vi "图像采集与保存-原版.vi"(9 "Grab":bool, 10 "保存图像":bool, 11 "Camera Name":refnum<k21>="cam0" caption="IMAQdx Session") -> ()   [LabVIEW 2018]
doc: "The Grab and Attributes Setup example VI allows the user to view the current attributes and settings, update attribute settings, acquire images continuously, and display the images in an image control."
uses:
  <vilib>/vision/driver/IMAQdx.llb/IMAQdx Acquisition Mode.ctl
  <vilib>/vision/driver/IMAQdx.llb/IMAQdx Buffer Number Mode.ctl
  <vilib>/vision/driver/NI_Vision_Acquisition_Software.lvlib
panel:
  in  "确定按钮":bool
  in  "Tab Control":T1(tab)
  in  "U32 Value Control":u32(slide) min=1 step=1 scale=1.0..4294967295.0
  in  "DBL Value Control":dbl(slide) min=2.2571161239684447 max=1000.0 step=1.0 scale=2.2571161239684447..1000.0
  in  "String Value Control":string
  in  "Enum Value Control":u32(ring) items=["Unicast", "Broadcast", "Multicast"]
  in  "Boolean Value Control":bool
  in  "Command Value Control":bool
  out "Tooltip":string="Gets/Sets the maximum number of outstanding events to queue."
  out "Units":string
  in  "Attribute Tree":string(tree)
  out "Frame Rate":dbl(knob) scale=0.0..100.0
  out "Image":T2(plugin-control)
  out "Buffer Number":u32
  in  "Stop":bool
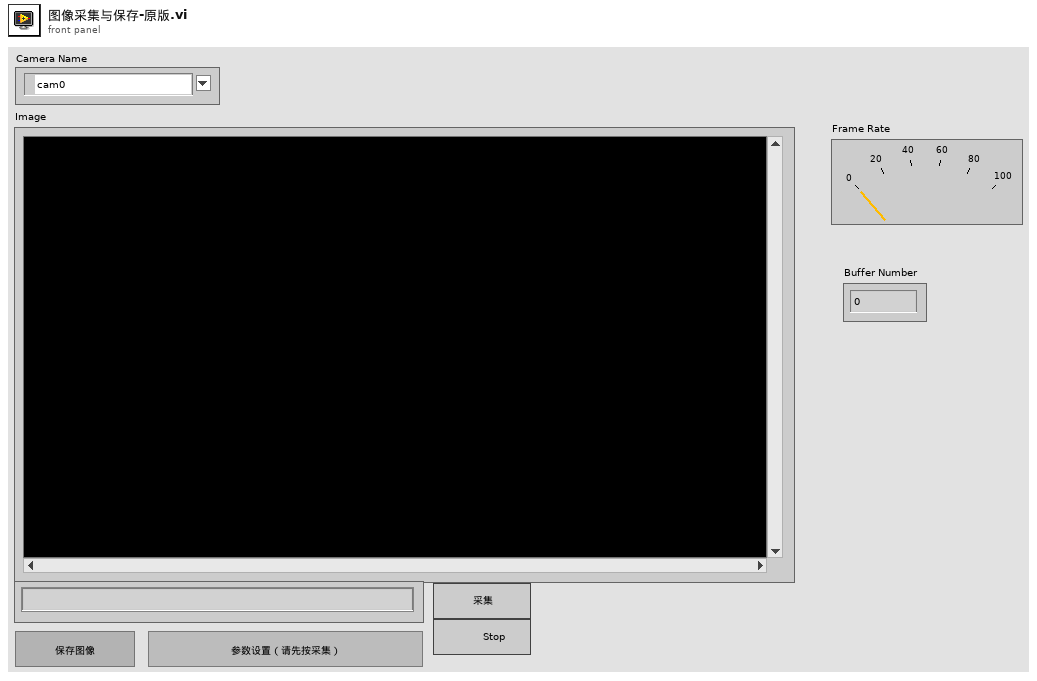
[diagram p1: front panel]
types:
  T1 = enum32{"U32", "DBL", "String", "Enum", "Bool", "Command"}
  T2 = typedef "IMAQ Image.ctl" = refnum<image>
  T3 = typedef "NI_Vision_Acquisition_Software.lvlib/IMAQdx Acquisition Mode.ctl" = enum32{"One Shot", "Continuous"}
  T4 = typedef "IMAQdx.ctl" = refnum<k21>
  T5 = cluster{"Tab Control":refnum<vi>, "U32 Value Control":refnum<vi>, "DBL Value Control":refnum<vi>, "String Value Control":refnum<vi>, "Enum Value Control":refnum<vi>, "Boolean Value Control":refnum<vi>, "Command Value Control":refnum<vi>}
  T6 = typedef "NI_Vision_Acquisition_Software.lvlib/IMAQdx Buffer Number Mode.ctl" = enum32{"Next", "Last", "Buffer Number", "Every", "Last New"}
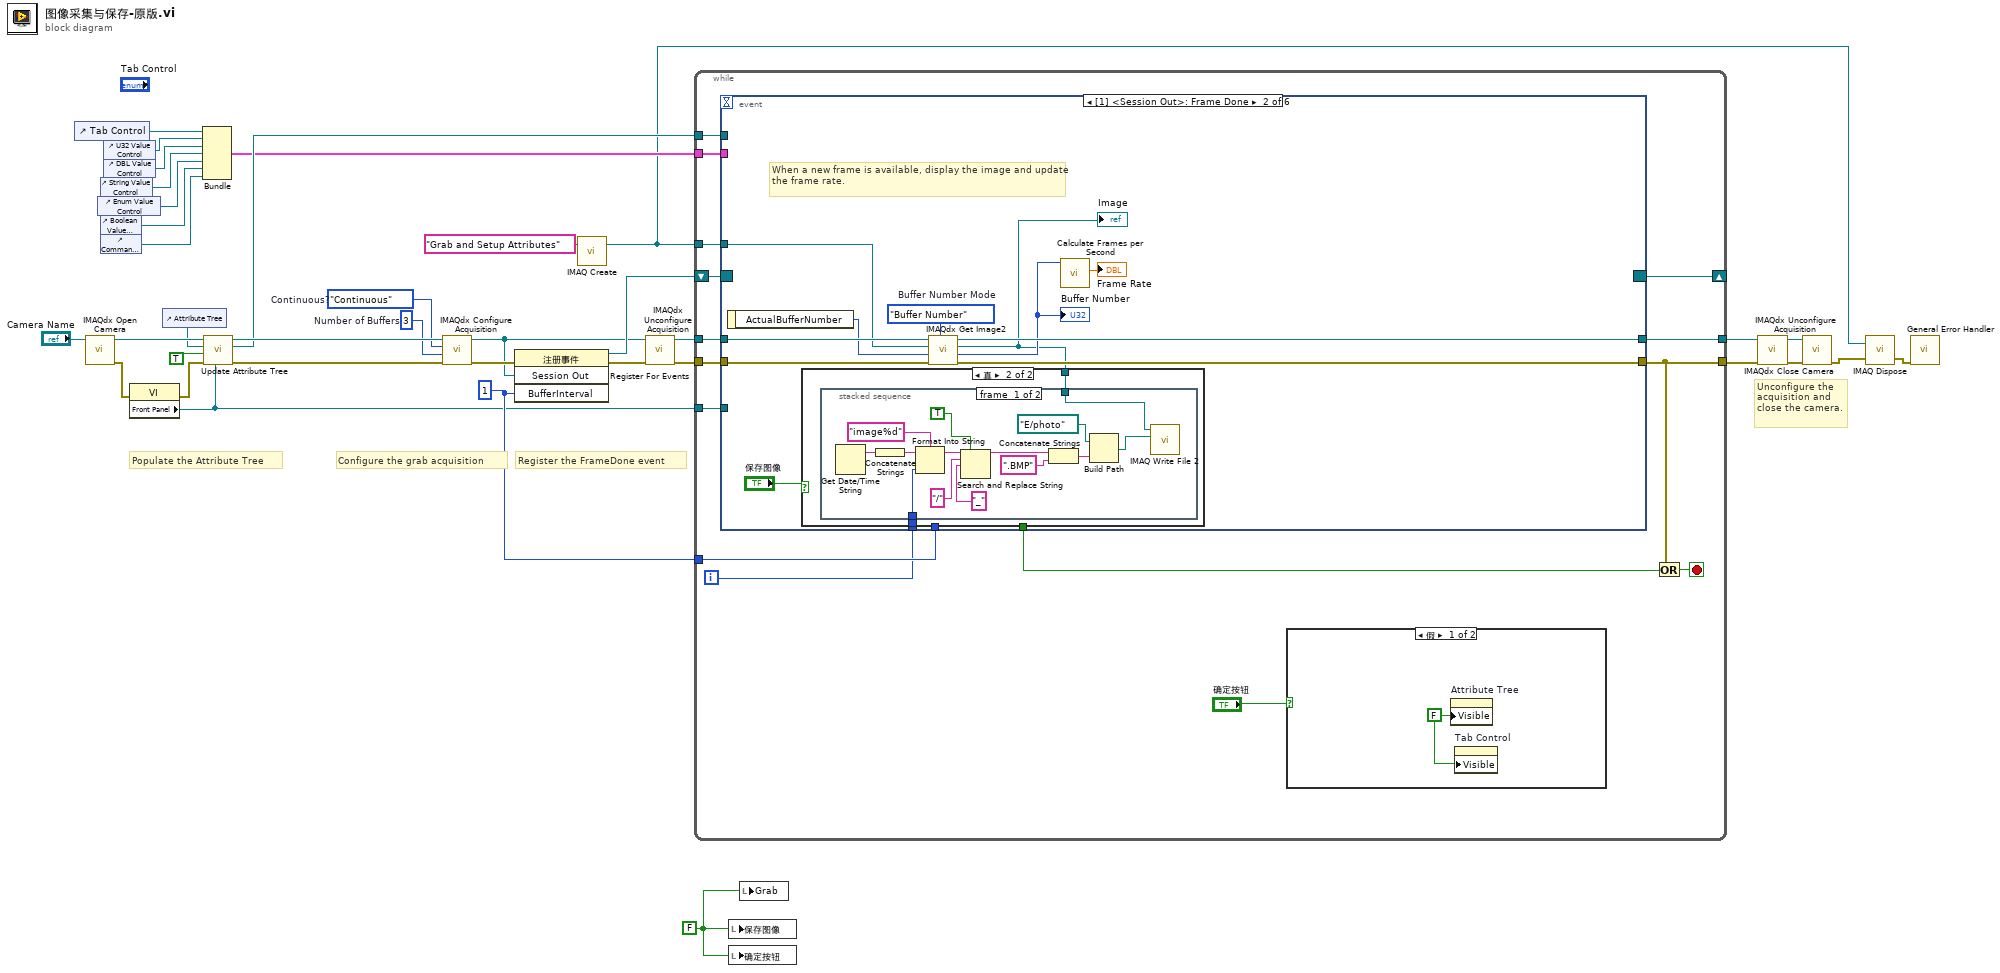
[diagram p0: block diagram]
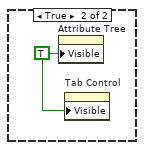
[diagram p2: hidden frame]
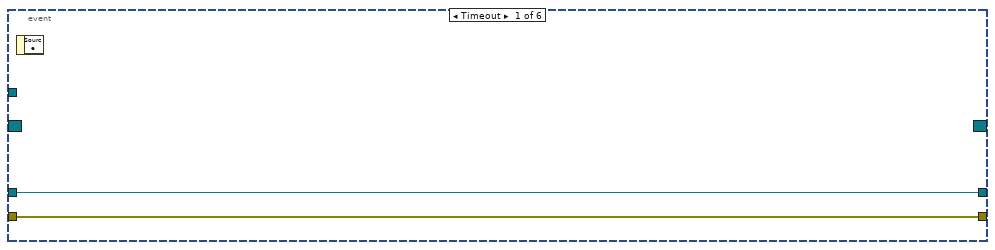
[diagram p3: hidden frame]
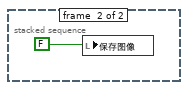
[diagram p5: hidden frame]
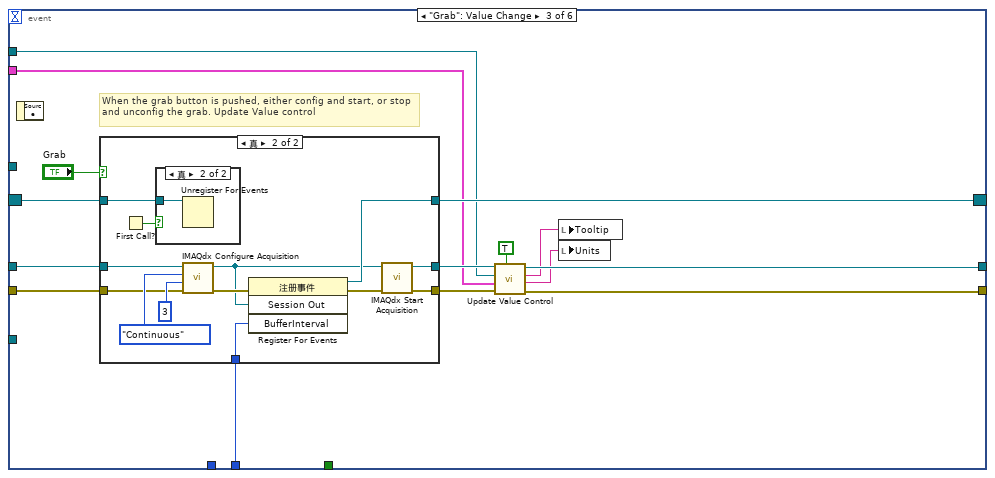
[diagram p6: hidden frame]
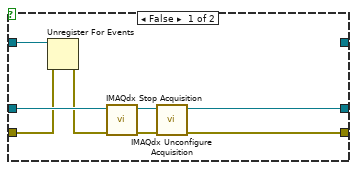
[diagram p7: hidden frame]
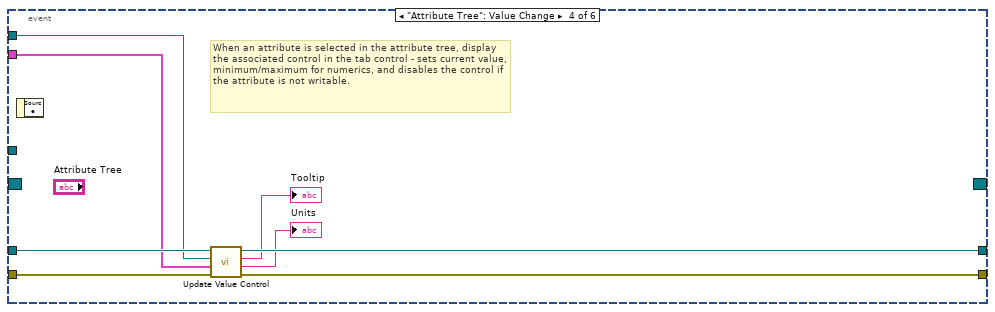
[diagram p9: hidden frame]
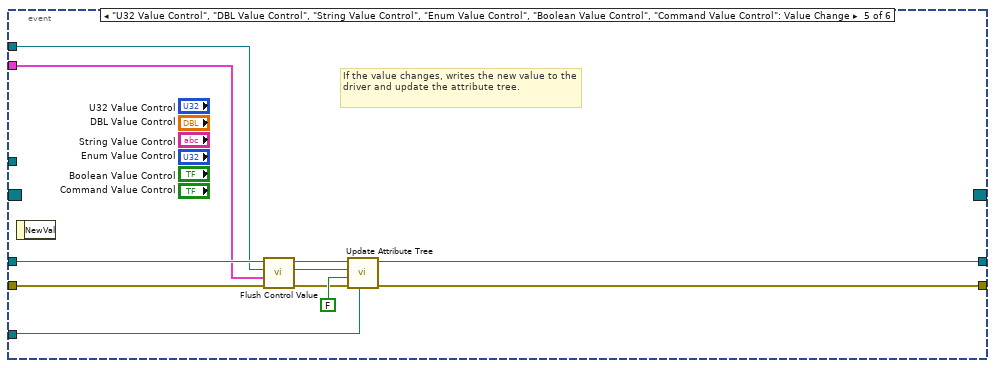
[diagram p10: hidden frame]
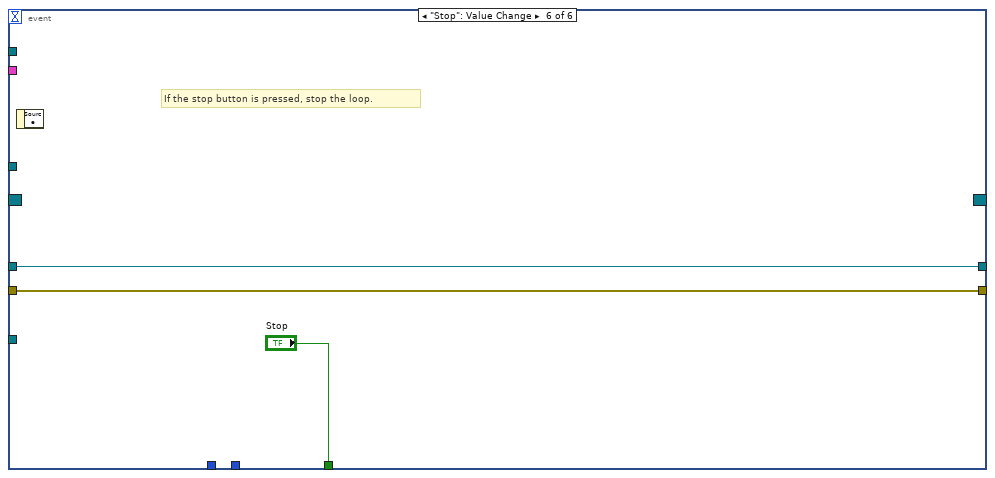
[diagram p11: hidden frame]
diagram:
  w1 = FALSE
  w17 = u32 1 ("BufferInterval")
  w3 = u32 3  # Number of Buffers
  w2 = IMAQdx_Acquisition_Mode."Continuous"  # Continuous?
  # "Unconfigure the acquisition and close the camera."
  # "Register the FrameDone event"
  # "Configure the grab acquisition"
  # "Populate the Attribute Tree"
  n1 = control-ref of="Tab Control"() -> (w7:refnum<vi>)
  n2 = call <vilib>:"IMAQdx Open Camera.vi"("Session In"="Camera Name") -> ("error out"=w20:errorcluster, "Session Out"=w25:T4)  [unwired: 2 in, 7 out]
  n3 = control-ref of="Enum Value Control"() -> (w28:refnum<vi>)
  n4 = control-ref of="String Value Control"() -> (w31:refnum<vi>)
  n5 = control-ref of="Boolean Value Control"() -> (w27:refnum<vi>)
  n6 = control-ref of="Command Value Control"() -> (w26:refnum<vi>)
  n7 = control-ref of="U32 Value Control"() -> (w30:refnum<vi>)
  n8 = control-ref of="DBL Value Control"() -> (w29:refnum<vi>)
  n9 = property class="VI"(error in=w20) -> (error out=w6:errorcluster, "Front Panel"=w4:refnum<vi>)  [unwired: 1 in, 1 out]
  n10 = control-ref of="Attribute Tree"() -> (w23:refnum<vi>)
  n11 = Bundle("Tab Control"=w7, "U32 Value Control"=w30, "DBL Value Control"=w29, "String Value Control"=w31, "Enum Value Control"=w28, "Boolean Value Control"=w27, "Command Value Control"=w26) -> (w12:T5)  [unwired: 1 out]
  n12 = call "Update Attribute Tree.vi"("Panel Refnum In"=w4, "error in"=w6, "Flush Tree?"=TRUE, "Tree Control In"=w23, "Camera Name In"=w25) -> ("error out"=w5:errorcluster, "Tree Control Out"=w21:refnum<vi>, "Session Out"=w24:T4)  [unwired: 4 in]
  n13 = call <vilib>:"IMAQdx Configure Acquisition.vi"("error in"=w5, "Number of Buffers"=w3, "Continuous?"=w2, "Session In"=w24) -> ("error out"=w33:errorcluster, "Session Out"=w14:T4)  [unwired: 6 out]
  n14 = register-events(error in=w33, w14, w17) -> (reference out=w32:refnum<event-registration>, error out=w16:errorcluster)  [unwired: 1 in]
  n15 = call "IMAQ Create"("Image Name"="Grab and Setup Attributes") -> ("New Image"=w9:T2)  [unwired: 3 in, 2 out]
  n16 = call <vilib>:"IMAQdx Unconfigure Acquisition.vi"("error in"=w16, "Session In"=w14) -> ("error out"=w15:errorcluster, "Session Out"=w13:T4)  [unwired: 8 out]
  n17 = while {
    tunnel: [w47] -> w19
    tunnel: w15 -> [w49]
    tunnel: w13 -> [w50]
    tunnel: [w40] -> w18
    tunnel: w9 -> [w48]
    tunnel: w21 -> [w45]
    tunnel: w4 -> [w44]
    tunnel: w17 -> [w42]
    shift-right: [w41] -> _
    shift-left: w32 -> [w46]
    tunnel: w12 -> [w39]
    i -> [w38]
    stop <- w51 stop-if-true
    n18 = event shown="[1] <Session Out>: Frame Done" {
      selector: w46 -> [_ _ w95 _ _ _]
      dyn-events: [_ _ w97 _ _ _] -> w41
      timeout: _ -> [_ _ _ _ _ _]
      tunnel: w50 -> [w54 w67 w99 w129 w139 w141]
      tunnel: w49 -> [w55 w66 w94 w127 w140 w142]
      tunnel: w48 -> [_ w65 _ _ _ _]
      tunnel: [w54 w64 w87 w128 w135 w141] -> w47
      tunnel: [w55 w63 w91 w126 w131 w142] -> w40
      tunnel: w45 -> [_ _ w90 w124 w133 _]
      tunnel: w44 -> [_ _ _ _ w130 _]
      tunnel: [_ _ _ _ _ "Stop"] -> w43
      tunnel: w42 -> [_ _ w96 _ _ _]
      tunnel: w39 -> [_ _ w88 w125 w134 _]
      tunnel: w38 -> [_ w57 _ _ _ _]
      event Timeout {
        n19 = event-data() -> ()  [unwired: 2 out]
      }
      event event #0x0 {
        w62 = IMAQdx_Buffer_Number_Mode."Buffer Number"  # Buffer Number Mode
        # "When a new frame is available, display the image and update the frame rate."
        n20 = event-data() -> ("ActualBufferNumber"=w61:u32)  [unwired: 1 out]
        n21 = call <vilib>:"IMAQdx Get Image2.vi"("Buffer Number Mode (Next)"=w62, "error in"=w66, "Buffer Number In"=w61, "Image In"=w65, "Session In"=w67) -> ("error out"=w63:errorcluster, "Buffer Number Out"=w60:u32, "Image Out"=w56:T2, "Session Out"=w64:T4)  [unwired: 3 in]
        "Image" <- w56
        "Buffer Number" <- w60
        n22 = case shown="真" "保存图像" {
          tunnel: w57 -> [_ w69]
          tunnel: w56 -> [_ w68]
          frame False {
          }
          frame True {
            n23 = stacked-sequence {
              tunnel: w69 -> [w71 _]
              tunnel: w68 -> [w70 _]
              frame #0 {
                n24 = Get Date/Time String() -> (date string=w75:string)  [unwired: 3 in, 1 out]
                n25 = Concatenate Strings(w75) -> (w74:string)
                n26 = Format Into String(format string="image%d" ("Image Name"), initial string=w74, w71) -> (resulting string=w72:string)  [unwired: 1 in, 1 out]
                n27 = Search and Replace String(replace all?=TRUE ("替换全部？(F)"), input string=w72, search string="/" ("搜索字符串"), replace string="_" ("替换字符串(\"\")")) -> (result string=w77:string)  [unwired: 4 in, 3 out]
                n28 = Concatenate Strings(w77, ".BMP" ("字符串")) -> (w76:string)
                n29 = Build Path(base path=path "E:/photo" ("基路径"), name or relative path=w76) -> (appended path=w83:path)
                n30 = call-poly "IMAQ Write File 2"("File Path"=w83, "Image"=w70) -> ()  [unwired: 8 in, 2 out]
              }
              frame #1 {
                n31 = local write "保存图像"(FALSE) -> ()
              }
            }
          }
        }
        n32 = call <vilib>:"Calculate Frames per Second.vi"("Buffer Number"=w60) -> ("Processed Frames/s"=→"Frame Rate":dbl)  [unwired: 8 in, 2 out]
      }
      event "Grab": Value Change {
        # "When the grab button is pushed, either config and start, or stop and unconfig the grab. Update Value control"
        n33 = event-data() -> ()  [unwired: 2 out]
        n34 = case shown="真" "Grab" {
          tunnel: w99 -> [w107 w118]
          tunnel: [w104 w120] -> w93
          tunnel: [w103 w119] -> w92
          tunnel: [_ w113] -> w97
          tunnel: w96 -> [_ w111]
          tunnel: w95 -> [w102 w109]
          tunnel: w94 -> [w100 w110]
          frame False {
            n35 = Unregister For Events(event registration refnum=w102, error in=w100) -> (error out=w101:errorcluster)
            n36 = call <vilib>:"IMAQdx Stop Acquisition.vi"("error in"=w101, "Session In"=w107) -> ("error out"=w105:errorcluster, "Session Out"=w106:T4)  [unwired: 8 out]
            n37 = call <vilib>:"IMAQdx Unconfigure Acquisition.vi"("error in"=w105, "Session In"=w106) -> ("error out"=w103:errorcluster, "Session Out"=w104:T4)  [unwired: 8 out]
          }
          frame True {
            n38 = First Call?() -> (First Call?: T/F=w108:bool)
            n39 = case shown="真" w108 {
              tunnel: w109 -> [_ w121]
              frame False {
              }
              frame True {
                n40 = Unregister For Events(event registration refnum=w121) -> ()  [unwired: 1 in, 1 out]
              }
            }
            n41 = call <vilib>:"IMAQdx Configure Acquisition.vi"("error in"=w110, "Number of Buffers"=u32 3, "Continuous?"=IMAQdx_Acquisition_Mode."Continuous", "Session In"=w118) -> ("error out"=w115:errorcluster, "Session Out"=w112:T4)  [unwired: 6 out]
            n42 = register-events(error in=w115, w112, w111) -> (reference out=w113:refnum<event-registration>, error out=w114:errorcluster)  [unwired: 1 in]
            n43 = call <vilib>:"IMAQdx Start Acquisition.vi"("error in"=w114, "Session In"=w112) -> ("error out"=w119:errorcluster, "Session Out"=w120:T4)  [unwired: 8 out]
          }
        }
        n44 = call "Update Value Control.vi"("Force update?"=TRUE, "error in (no error)"=w92, "Tab Control Ref In"=w88, "Tree Control In"=w90, "Session In"=w93) -> ("error out"=w91:errorcluster, "Units"=w85:string, "Tooltip"=w86:string, "Session Out"=w87:T4)  [unwired: 3 in]
        n45 = local write "Tooltip"(w86) -> ()
        n46 = local write "Units"(w85) -> ()
      }
      event "Attribute Tree": Value Change {
        # "When an attribute is selected in the attribute tree, display the associated control in the tab control - sets current value, minimum/maximum for numerics, and disables the control if the attribute is not writable."
        n47 = event-data() -> ()  [unwired: 2 out]
        n48 = call "Update Value Control.vi"("error in (no error)"=w127, "Tab Control Ref In"=w125, "Tree Control In"=w124, "Session In"=w129) -> ("error out"=w126:errorcluster, "Units"=→"Units":string, "Tooltip"=→"Tooltip":string, "Session Out"=w128:T4)  [unwired: 4 in]
      }
      event "U32 Value Control", "DBL Value Control", "String Value Control", "Enum Value Control", "Boolean Value Control", "Command Value Control": Value Change {
        # "If the value changes, writes the new value to the driver and update the attribute tree."
        n49 = event-data() -> ()  [unwired: 2 out]
        n50 = call "Flush Control Value.vi"("error in (no error)"=w140, "Tab Control Ref In"=w134, "Tree Control In"=w133, "Session In"=w139) -> ("error out"=w132:errorcluster, "Tree Control Out"=w137:refnum<vi>, "Session Out"=w138:T4)  [unwired: 5 in]
        n51 = call "Update Attribute Tree.vi"("Panel Refnum In"=w130, "error in"=w132, "Flush Tree?"=FALSE, "Tree Control In"=w137, "Camera Name In"=w138) -> ("error out"=w131:errorcluster, "Session Out"=w135:T4)  [unwired: 4 in, 1 out]
      }
      event "Stop": Value Change {
        # "If the stop button is pressed, stop the loop."
        n52 = event-data() -> ()  [unwired: 2 out]
      }
    }
    n53 = case shown="假" "确定按钮" {
      frame False {
        w52 = FALSE ("可见")
        n54 = property on="Attribute Tree" class="Tree (严格)"("Visible"=w52) -> ()  [unwired: 2 in, 2 out]
        n55 = property on="Tab Control" class="TabCtl (严格)"("Visible"=w52) -> ()  [unwired: 2 in, 2 out]
      }
      frame True {
        w53 = TRUE ("可见")
        n56 = property on="Attribute Tree" class="Tree (严格)"("Visible"=w53) -> ()  [unwired: 2 in, 2 out]
        n57 = property on="Tab Control" class="TabCtl (严格)"("Visible"=w53) -> ()  [unwired: 2 in, 2 out]
      }
    }
    n58 = Or(x=w40, y=w43) -> (x .or. y?=w51:bool)
  }
  n59 = local write "保存图像"(w1) -> ()
  n60 = local write "确定按钮"(w1) -> ()
  n61 = local write "Grab"(w1) -> ()
  n62 = call <vilib>:"IMAQdx Unconfigure Acquisition.vi"("error in"=w18, "Session In"=w19) -> ("error out"=w35:errorcluster, "Session Out"=w34:T4)  [unwired: 8 out]
  n63 = call <vilib>:"IMAQdx Close Camera.vi"("error in"=w35, "Session In"=w34) -> ("error out"=w11:errorcluster)  [unwired: 9 out]
  n64 = call "IMAQ Dispose"("Image"=w9, "error in (no error)"=w11) -> ("error out"=w10:errorcluster)  [unwired: 4 in]
  n65 = call <vilib>:"General Error Handler.vi"("error in (no error)"=w10) -> ()  [unwired: 2 in, 13 out]
